vi "Write Mode.vi"(8 "error in (no error)":errorcluster, 10 "Mode":T1, 11 "String Compare in":refnum<class "String Compare.lvclass">) -> (0 "error out":errorcluster, 3 "String Compare out":refnum<class "String Compare.lvclass">)   [LabVIEW 2015, in "String Compare.lvclass"]
uses:
  String Compare.lvclass
  Config/Mode.ctl
  String Compare.lvclass/String Compare.ctl
  Config/String Compare Config.lvclass
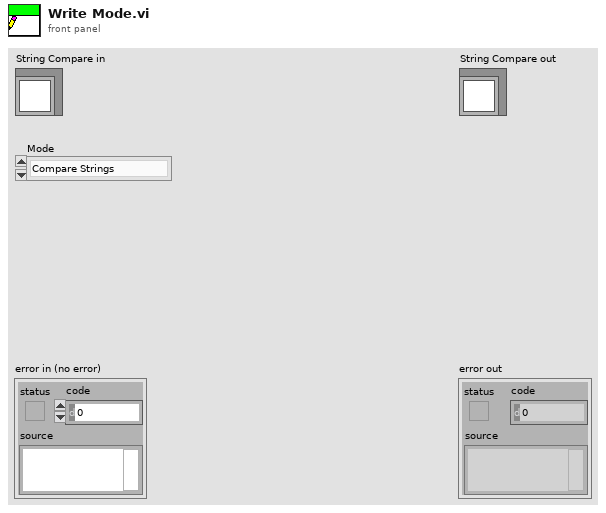
[diagram p1: front panel]
types:
  T1 = typedef "String Compare Config.lvclass/Mode.ctl" = enum16{"Compare Strings", "Match Regex"}
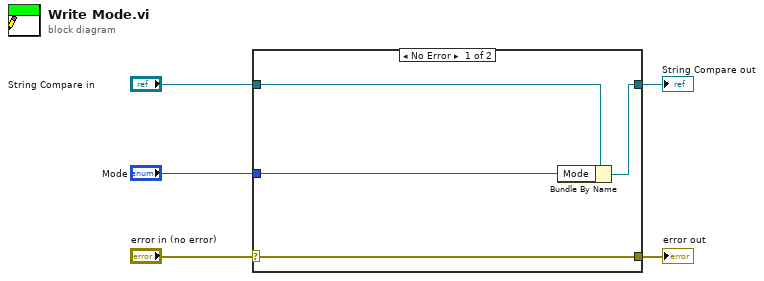
[diagram p0: block diagram]
diagram:
  n1 = case shown="No Error" "error in (no error)" {
    selector: "error in (no error)" -> [w9 w10]
    tunnel: [w9 w10] -> w4
    tunnel: [w7 w11] -> w2
    tunnel: "String Compare in" -> [w8 w11]
    tunnel: "Mode" -> [w6 _]
    frame No Error {
      n2 = Bundle By Name(cluster=w8, "Mode"=w6) -> (w7:refnum<class "String Compare.lvclass">)
    }
    frame Error {
    }
  }
  "error out" <- w4
  "String Compare out" <- w2
